vi "qmh_example.vi"() -> ()   [LabVIEW 2020]
uses:
  main_ref.ctl
  message.ctl
  states.ctl
  <vilib>/addons/zeromq/zmq_socket.lvclass
panel:
  in  "Temperature setpoint":dbl
  out "Temperature Chart":dbl(graph)
  out "error out":errorcluster
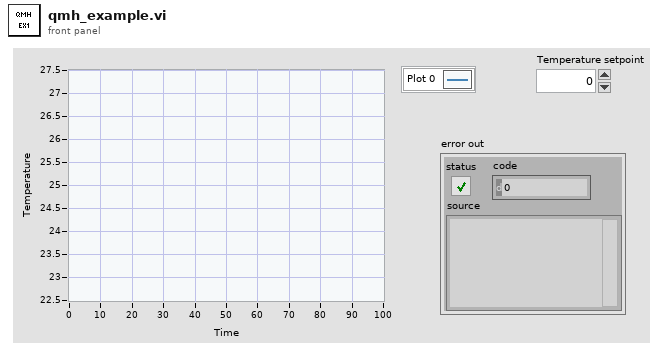
[diagram p1: front panel]
types:
  T1 = typedef "main_ref.ctl" = cluster{"messageHandlerQ":refnum<queue>, "stopEvent":refnum<user-event>}
  T2 = typedef "states.ctl" = enum16{"update temperature (API)", "update temperature (User)", "stop"}
  T3 = typedef "message.ctl" = cluster{"states":T2, "Payload":variant}
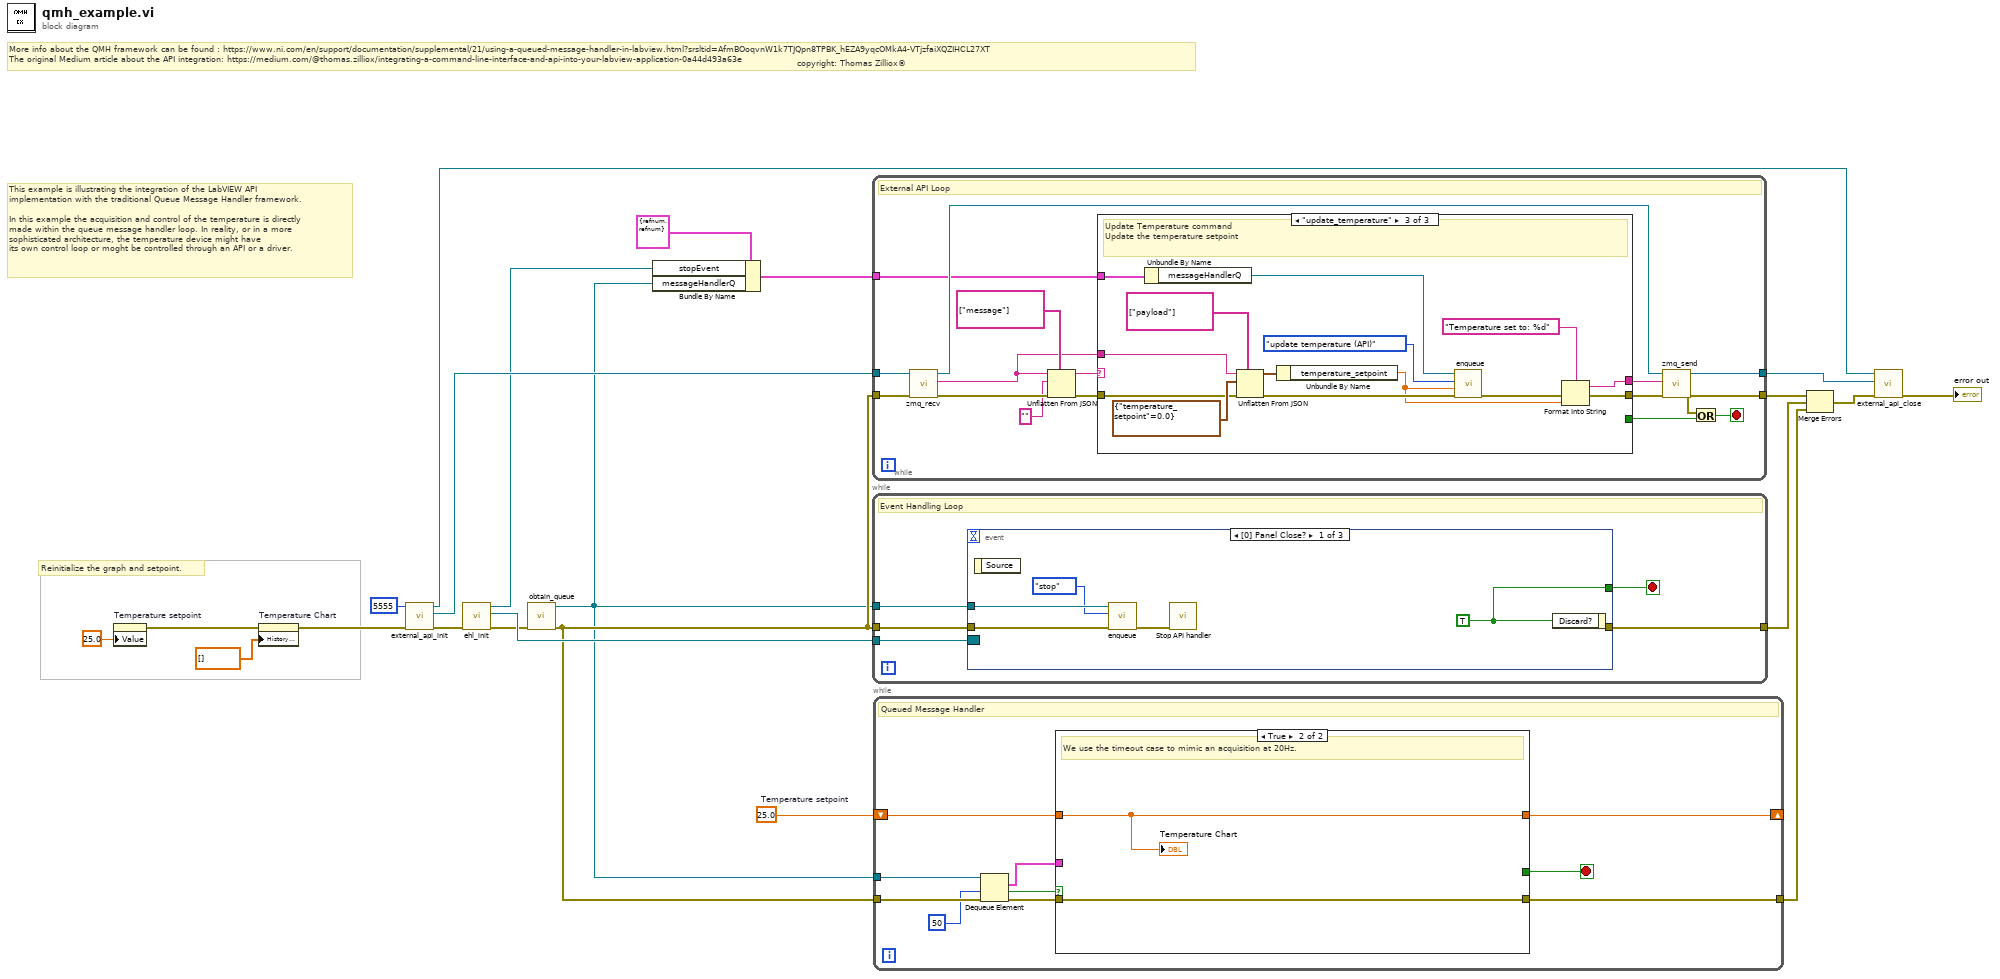
[diagram p0: block diagram]
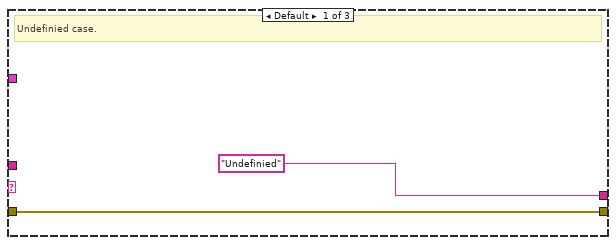
[diagram p2: hidden frame]
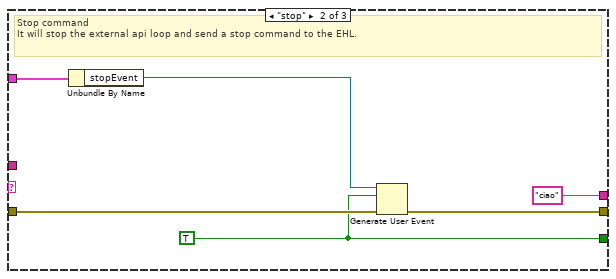
[diagram p3: hidden frame]
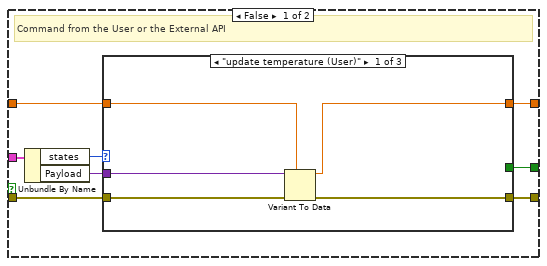
[diagram p4: hidden frame]
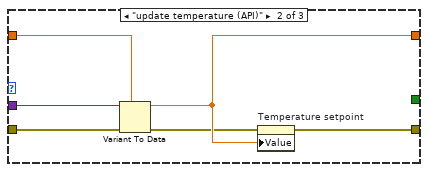
[diagram p5: hidden frame]
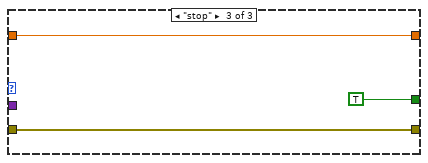
[diagram p6: hidden frame]
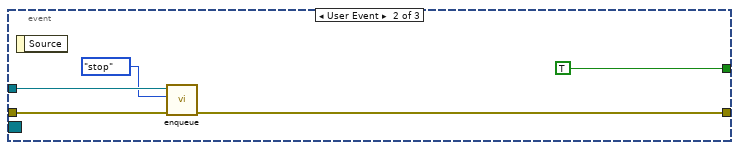
[diagram p7: hidden frame]
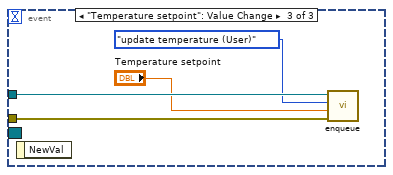
[diagram p8: hidden frame]
diagram:
  w15 = 25.0  # Temperature setpoint
  # "More info about the QMH framework can be found : https://www.ni.com/en/support/documentation/supplemental/21/using-a-queued-message-handler-in-labview.html?srsltid=AfmBOoqvnW1k7TJQpn8TPBK_hEZA9yqcOMkA4-VTjzfaiXQZIHCL27XT\nThe original Medium article about the API integration: https://medium.com/@thomas.zilliox/integrating-a-command-line-interface-and-api-into-your-labview-application-0a44d493a63e"
  # "This example is illustrating the integration of the LabVIEW API\nimplementation with the traditional Queue Message Handler framework.\n\nIn this example the acquisition and control of the temperature is directly\nmade within the queue message handler loop. In reality, or in a more \nsophisticated architecture, the temperature device might have\nits own control loop or moght be controlled through an API or a driver."
  # "Reinitialize the graph and setpoint."
  # "copyright: Thomas Zilliox©"
  n1 = property on="Temperature setpoint" class="DigNum (strict)"("Value"=25.0 ("Temperature setpoint")) -> (error out=w14:errorcluster)  [unwired: 2 in, 1 out]
  n2 = property on="Temperature Chart" class="WFChart (strict)"(error in=w14, "History Data"=dbl[] []) -> (error out=w12:errorcluster)  [unwired: 1 in, 1 out]
  n3 = call "external_api_init.vi"("error in (no error)"=w12, "Port (5555)"=5555) -> ("error out"=w10:errorcluster, "socket out"=w19:refnum<class "zmq_socket.lvclass">, "zmq_context out"=w20:refnum<class "zmq_context.lvclass">)  [unwired: 7 in]
  n4 = call "ehl_init.vi"("error in (no error)"=w10) -> ("error out"=w9:errorcluster, "Event Registration Refnum"=w11:refnum<event-registration>, "User Event out"=w3:refnum<user-event>)  [unwired: 8 in]
  n5 = call "obtain_queue.vi"("error in (no error)"=w9) -> ("error out"=w8:errorcluster, "queue out"=w2:refnum<queue>)  [unwired: 9 in]
  n6 = Bundle By Name(cluster=T1 {"messageHandlerQ"=refnum, "stopEvent"=refnum} ("Cluster"), "stopEvent"=w3, "messageHandlerQ"=w2) -> (w1:T1)
  n7 = while {
    tunnel: w19 -> [w38]
    tunnel: w8 -> [w37]
    tunnel: [w35] -> w18
    tunnel: [w34] -> w17
    tunnel: w1 -> [w23]
    stop <- w33 stop-if-true
    # "External API Loop"
    n8 = call <vilib>:"zmq_recv.vi"("error in"=w37, "socket in"=w38) -> ("error out"=w30:errorcluster, "data"=w25:string, "socket out"=w36:refnum<class "zmq_socket.lvclass">)  [unwired: 3 in, 2 out]
    n9 = Unflatten From JSON(path=string[] ["message"], JSON string=w25, type and defaults="", error in (no error)=w30) -> (value=w27:string, error out=w29:errorcluster)  [unwired: 3 in]
    n10 = case shown="\"update_temperature\"" w27 {
      tunnel: [w40 w44 w60] -> w32
      tunnel: w29 -> [w40 w46 w55]
      tunnel: [_ w43 _] -> w31
      tunnel: ["Undefinied" ("data") "ciao" ("data") w58] -> w24
      tunnel: w25 -> [_ _ w52]
      tunnel: w23 -> [_ w42 w48]
      frame Default {
        # "Undefinied case."
      }
      frame "stop" {
        w43 = TRUE
        # "Stop command\nIt will stop the external api loop and send a stop command to the EHL."
        n11 = Unbundle By Name(w42) -> ("stopEvent"=w41:refnum<user-event>)
        n12 = Generate User Event(user event=w41, event data cluster=w43, error in=w46) -> (error out=w44:errorcluster)  [unwired: 1 in, 1 out]
      }
      frame "update_temperature" {
        # "Update Temperature command\nUpdate the temperature setpoint"
        n13 = Unbundle By Name(w48) -> ("messageHandlerQ"=w47:refnum<queue>)
        n14 = Unflatten From JSON(path=string[] ["payload"], JSON string=w52, type and defaults=cluster{"temperature_setpoint":dbl} {"temperature_setpoint"=0.0}, error in (no error)=w55) -> (value=w53:cluster{"temperature_setpoint":dbl}, error out=w54:errorcluster)  [unwired: 3 in]
        n15 = Unbundle By Name(w53) -> ("temperature_setpoint"=w49:dbl)
        n16 = call "enqueue.vi"("error in (no error)"=w54, "Payload"=w49, "states"=states."update temperature (API)", "queue out"=w47) -> ("error out"=w51:errorcluster)  [unwired: 7 in]
        n17 = Format Into String(format string="Temperature set to: %d" ("data"), error in=w51, w49) -> (resulting string=w58:string, error out=w60:errorcluster)  [unwired: 1 in]
      }
    }
    n18 = call <vilib>:"zmq_send.vi"("error in"=w32, "data"=w24, "socket in"=w36) -> ("error out"=w34:errorcluster, "socket out"=w35:refnum<class "zmq_socket.lvclass">)  [unwired: 4 in]
    n19 = Or(x=w34, y=w31) -> (x .or. y?=w33:bool)
  }
  n20 = while {
    tunnel: w8 -> [w64]
    tunnel: w2 -> [w63]
    tunnel: w11 -> [w62]
    tunnel: [w61] -> w6
    stop <- w65 stop-if-true
    # "Event Handling Loop"
    n21 = event shown="[0] Panel Close?" {
      selector: w62 -> [_ _ _]
      dyn-events: _ -> [_ _ _]
      timeout: _ -> [_ _ _]
      tunnel: [w70 TRUE _] -> w65
      tunnel: w64 -> [w68 w73 w78]
      tunnel: w63 -> [w69 w74 w79]
      tunnel: [_ w71 _] -> w61
      event Panel Close? {
        w70 = TRUE
        n22 = event-data() -> ()  [unwired: 1 in, 1 out]
        n23 = call "enqueue.vi"("error in (no error)"=w68, "states"=states."stop", "queue out"=w69) -> ("error out"=w66:errorcluster)  [unwired: 8 in]
        n24 = call "Stop API handler.vi"("error in (no error)"=w66) -> ()  [unwired: 10 in, 1 out]
        n25 = event-data("Discard?"=w70) -> ()  [unwired: 1 in, 1 out]
      }
      event User Event {
        n26 = event-data() -> ()  [unwired: 1 in, 1 out]
        n27 = call "enqueue.vi"("error in (no error)"=w73, "states"=states."stop", "queue out"=w74) -> ("error out"=w71:errorcluster)  [unwired: 8 in]
      }
      event "Temperature setpoint": Value Change {
        n28 = event-data() -> ()  [unwired: 1 in, 1 out]
        n29 = call "enqueue.vi"("error in (no error)"=w78, "Payload"="Temperature setpoint", "states"=states."update temperature (User)", "queue out"=w79) -> ()  [unwired: 7 in, 1 out]
      }
    }
  }
  n30 = while {
    tunnel: w2 -> [w89]
    tunnel: w8 -> [w88]
    shift-right: [w81] -> _
    shift-left: w15 -> [w82]
    tunnel: [w80] -> w5
    stop <- w83 stop-if-true
    # "Queued Message Handler"
    n31 = Dequeue Element(queue=w89, timeout in ms (-1)=50, error in (no error)=w88) -> (element=w84:T3, timed out?=w86:bool, error out=w87:errorcluster)  [unwired: 1 out]
    n32 = case shown="True" w86 {
      tunnel: w87 -> [w96 w113]
      tunnel: w84 -> [w97 _]
      tunnel: [w94 _] -> w83
      tunnel: w82 -> [w93 w112]
      tunnel: [w92 w113] -> w80
      tunnel: [w90 w112] -> w81
      frame False {
        # "Command from the User or the External API"
        n33 = Unbundle By Name(w97) -> ("states"=w95:T2, "Payload"=w91:variant)
        n34 = case shown="\"update temperature (User)\"" w95 {
          tunnel: w96 -> [w102 w108 w110]
          tunnel: [_ _ TRUE] -> w94
          tunnel: w93 -> [w99 w106 w109]
          tunnel: [w101 w103 w110] -> w92
          tunnel: w91 -> [w100 w107 _]
          tunnel: [w98 w105 w109] -> w90
          frame "update temperature (User)" {
            n35 = Variant To Data(error in=w102, type=w99, Variant=w100) -> (data=w98:dbl, error out=w101:errorcluster)
          }
          frame "update temperature (API)" {
            n36 = Variant To Data(error in=w108, type=w106, Variant=w107) -> (data=w105:dbl, error out=w104:errorcluster)
            n37 = property on="Temperature setpoint" class="DigNum (strict)"(error in=w104, "Value"=w105) -> (error out=w103:errorcluster)  [unwired: 1 in, 1 out]
          }
          frame "stop" {
          }
        }
      }
      frame True {
        # "We use the timeout case to mimic an acquisition at 20Hz."
        "Temperature Chart" <- w112
      }
    }
  }
  n38 = Merge Errors(w17, w6, w5) -> (w7:errorcluster)
  n39 = call "external_api_close.vi"("error in (no error)"=w7, "socket in"=w18, "zmq_context in"=w20) -> ("error out"=→"error out":errorcluster)  [unwired: 8 in]
